vi "Stop Core.vi"(10 "final error code":i32, 11 "MFC in":refnum<class "Sensor & Control.lvclass">) -> (3 "MFC out":refnum<class "Sensor & Control.lvclass">)   [LabVIEW 2013, in "Sensor & Control.lvlib" / "Sensor & Control.lvclass"]
doc: "(<B>Filename</B>: Actor Framework.lvlib:Actor.lvclass:Stop Core.vi)\n\nDefines what the actor does before it stops. Use the <B>final error code</B> input to determine whether the actor shut down in response to an error.\n\nBy default, this method does nothing. A descendant class may override it to define behavior, such as shutting down any processes the actor initiated in its override of the Actor Core method."
uses:
  Sensor & Control.lvclass
  <vilib>/Instr/_visa.llb/VISA Flush IO Buffer Mask.ctl
  Sensor & Control.lvclass/Sensor & Control.ctl
  PluginInterface/PluginInterface.lvlibp/PluginInterfaceClass/PluginInterface.lvclass
  Read VISA.vi
  PluginInterface/PluginInterface.lvlibp/PluginInterfaceClass/Read TDMS.vi
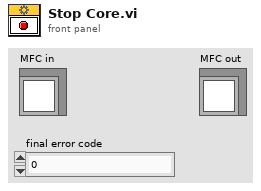
[diagram p1: front panel]
types:
  T1 = typedef "VISA Flush IO Buffer Mask.ctl" = u16
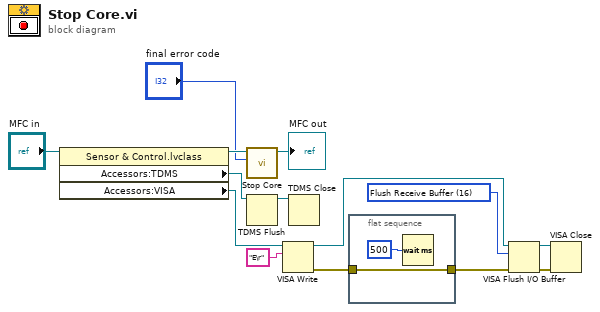
[diagram p0: block diagram]
diagram:
  w4 = T1 16 items=["Flush Receive Buffer"=16, "Write Transmit Buffer to Device"=32, "Flush Receive Buffer (No I/O)"=64, "Flush Transmit Buffer"=128] ("Mask")
  n1 = property class="Sensor & Control.lvclass"(reference="MFC in") -> (reference out=w14:refnum<class "Sensor & Control.lvclass">, "Accessors:TDMS"=w13:refnum<k34>, "Accessors:VISA"=w1:refnum<visa-resource-name>)  [unwired: 1 in, 1 out]
  n2 = call-parent "Stop Core.vi"("final error code"="final error code", "Actor in"=w14) -> ("Actor out"=→"MFC out":refnum<class "Sensor & Control.lvclass">)  [unwired: 9 in]
  n3 = TDMS Flush(7:w13) -> (3:w9:refnum<k34>)  [unwired: 1 in, 1 out]
  n4 = VISA Write(VISA resource name=w1, write buffer="E\r") -> (VISA resource name out=w5:refnum<visa-resource-name>, error out=w8:errorcluster)  [unwired: 1 in, 1 out]
  n5 = TDMS Close(11:w9) -> ()  [unwired: 1 in, 2 out]
  n6 = flat-sequence {
    tunnel: [w15] -> w6
    tunnel: w8 -> [w15]
    frame #0 {
      n7 = Wait (ms)(milliseconds to wait=u32 500) -> ()  [unwired: 1 out]
    }
  }
  n8 = VISA Flush I/O Buffer(VISA resource name=w5, mask (16)=w4, error in (no error)=w6) -> (VISA resource name out=w2:refnum<visa-resource-name>, error out=w3:errorcluster)
  n9 = VISA Close(VISA resource name=w2, error in (no error)=w3) -> ()  [unwired: 1 out]
